vi "AlazarCoprocessorRegisterWrite.vi"(3 "error in (no error)":errorcluster, 4 "Value":u32, 5 "Offset":u32, 6 "Handle":u64) -> (0 "error out":errorcluster, 1 "Return Code":u32, 2 "Handle":u64)   [LabVIEW 2018]
doc: "Write a value to a user-programmable coprocessor FPGA register."
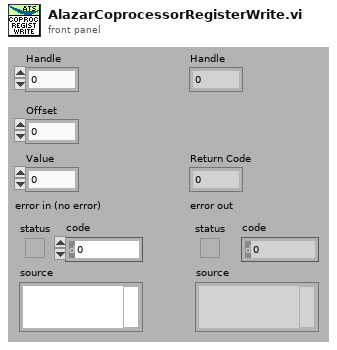
[diagram p1: front panel]
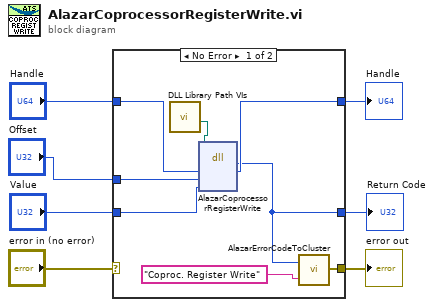
[diagram p0: block diagram]
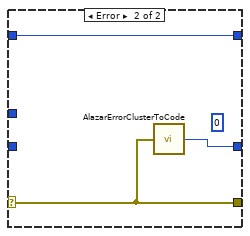
[diagram p2: hidden frame]
diagram:
  n1 = case shown="No Error" "error in (no error)" {
    selector: "error in (no error)" -> [_ w18]
    tunnel: [w11 w18] -> w6
    tunnel: [w10 w17] -> w5
    tunnel: "Handle" -> [w15 w16]
    tunnel: [w14 w16] -> w3
    tunnel: "Offset" -> [w13 _]
    tunnel: "Value" -> [w12 _]
    frame No Error {
      n2 = call "DLL Library Path VIs.vi"() -> ("Alazar"=w8:path)  [unwired: 9 in, 2 out]
      n3 = dll-call lib="C:/Project/SerialSectOCT - FFT GPU/SerialSectOCT/Labview Software/DLL/ATSApi.dll" fn="AlazarCoprocessorRegisterWrite"(path in=w8, "handle"=w15, "offset"=w13, "value"=w12) -> ("return type"=w10:u32, "handle"=w14:u64)  [unwired: 4 in, 2 out]
      n4 = call "AlazarErrorCodeToCluster.vi"("Message"="Coproc. Register Write", "Error Code"=w10) -> ("error out"=w11:errorcluster)
    }
    frame Error {
      (unwired) u32 0
      n5 = call "AlazarErrorClusterToCode.vi"("error in (no error)"=w18) -> ("Error Code"=w17:u32)
    }
  }
  "Handle" <- w3
  "error out" <- w6
  "Return Code" <- w5
